vi "LL_DELETE Object (Core).vi"(6 "Use HTTPS?":bool, 8 "error in (no error)":errorcluster, 9 "Bucket":string, 10 "Path and query string":string="/", 11 "Headers":T1[](array[typedef])) -> (0 "error out":errorcluster, 1 "Call Result":T2, 2 "Response body":string, 3 "Response header":string)   [LabVIEW 2011, in "LV Interface for Amazon S3.lvlib"]
doc: "This core implementation of the DELETE operation may be used to implement special requests or API calls not present in this toolkit."
uses:
  LV Interface for Amazon S3.lvlib
  Typedefs/AMZ_S3_Call Results.ctl
  Typedefs/AMZ_S3_HTTP Header-Value pair.ctl
  <vilib>/httpClient/LabVIEWHTTPClient.lvlib
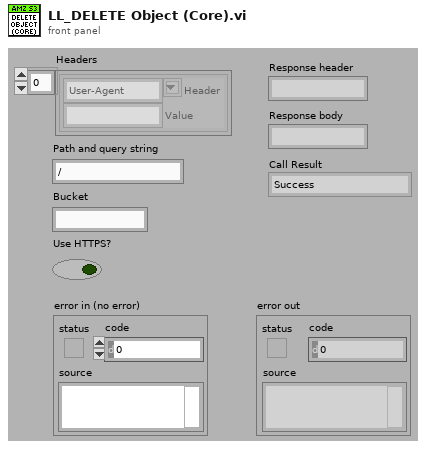
[diagram p1: front panel]
types:
  T1 = typedef "LV Interface for Amazon S3.lvlib/AMZ_S3_HTTP Header-Value pair.ctl" = cluster{"Header":string, "Value":string}
  T2 = typedef "LV Interface for Amazon S3.lvlib/AMZ_S3_Call Results.ctl" = enum16{"Success", "UndefinedError", "AccessDenied", "AccountProblem", "AmbiguousGrantByEmailAddress", "BadDigest", "BucketAlreadyExists", "BucketAlreadyOwnedByYou", "BucketNotEmpty", "CredentialsNotSupported", "CrossLocationLoggingProhibited", "EntityTooSmall", "EntityTooLarge", "ExpiredToken", "IllegalVersioningConfigurationException", "IncompleteBody", "IncorrectNumberOfFilesInPostRequest", "InlineDataTooLarge", "InternalError", "InvalidAccessKeyId", "InvalidAddressingHeader", "InvalidArgument", "InvalidBucketName", "InvalidDigest", "InvalidLocationConstraint", "InvalidPart", "InvalidPartOrder", "InvalidPayer", "InvalidPolicyDocument", "InvalidRange", "InvalidSecurity", "InvalidSOAPRequest", "InvalidStorageClass", "InvalidTargetBucketForLogging", "InvalidToken", "InvalidURI", "KeyTooLong", "MalformedACLError", "MalformedPOSTRequest", "MalformedXML", "MaxMessageLengthExceeded", "MaxPostPreDataLengthExceededError", "MetadataTooLarge", "MethodNotAllowed", "MissingAttachment", "MissingContentLength", "MissingRequestBodyError", "MissingSecurityElement", "MissingSecurityHeader", "NoLoggingStatusForKey", "NoSuchBucket", "NoSuchKey", "NoSuchUpload", "NoSuchVersion", "NotImplemented", "NotSignedUp", "OperationAborted", "PermanentRedirect", "PreconditionFailed", "Redirect", "RequestIsNotMultiPartContent", "RequestTimeout", "RequestTimeTooSkewed", "RequestTorrentOfBucketError", "SignatureDoesNotMatch", "SlowDown", "TemporaryRedirect", "TokenRefreshRequired", "TooManyBuckets", "UnexpectedContent", "UnresolvableGrantByEmailAddress", "UserKeyMustBeSpecified", "LabVIEWError"}
  T3 = typedef "LabVIEWHTTPClient.lvlib/ClientHandle.ctl" = refnum<k1>
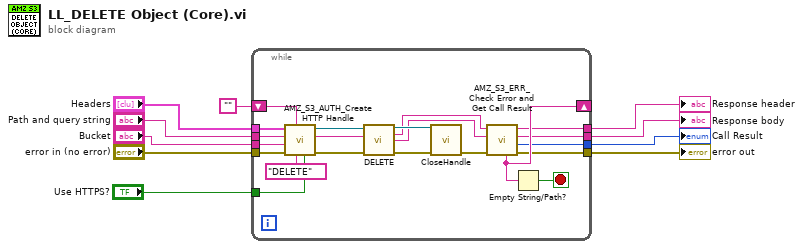
[diagram p0: block diagram]
diagram:
  n1 = while {
    tunnel: "error in (no error)" -> [w30]
    tunnel: "Bucket" -> [w29]
    tunnel: "Path and query string" -> [w28]
    tunnel: "Headers" -> [w27]
    shift-right: [w16] -> _
    shift-left: "" -> [w26]
    tunnel: [w15] -> w9
    tunnel: [w14] -> w8
    tunnel: [w13] -> w3
    tunnel: [w12] -> w2
    tunnel: "Use HTTPS?" -> [w11]
    stop <- w17 stop-if-true
    n2 = call "AMZ_S3_AUTH_Create HTTP Handle.vi"("Use HTTPS?"=w11, "HTTP-Verb"="DELETE", "Redirect endpoint"=w26, "error in (no error)"=w30, "Bucket"=w29, "Path and query string"=w28, "Headers"=w27) -> ("error out"=w25:errorcluster, "URL"=w24:string, "client handle out"=w23:T3)  [unwired: 2 in]
    n3 = call <vilib>:"DELETE.vi"("client handle"=w23, "url"=w24, "error in (no error)"=w25) -> ("client handle out"=w22:T3, "headers"=w19:string, "body"=w18:string, "error out"=w21:errorcluster)  [unwired: 9 in]
    n4 = call <vilib>:"CloseHandle.vi"("client handle"=w22, "error in (no error)"=w21) -> ("error out"=w20:errorcluster)  [unwired: 13 in]
    n5 = call "AMZ_S3_ERR_Check Error and Get Call Result.vi"("error in (no error)"=w20, "Response body"=w18, "Response header"=w19) -> ("error out"=w15:errorcluster, "Call Result"=w14:T2, "Response body dup"=w13:string, "Response header dup"=w12:string, "Redirect endpoint"=w16:string)  [unwired: 4 in]
    n6 = Empty String/Path?(string/path=w16) -> (empty?=w17:bool)
  }
  "error out" <- w9
  "Call Result" <- w8
  "Response body" <- w3
  "Response header" <- w2
